vi "ExitApp (SubVI).vi"(8 "error in (no error)":errorcluster, 11 "Display Queue in":refnum<queue>) -> (0 "error out":errorcluster, 3 "Display Queue out":refnum<queue>)   [LabVIEW 2017]
uses:
  Controls/DisplayControl.ctl
  Controls/DisplayCommand.ctl
  Controls/UpdateMessageControl.ctl
  Controls/UpdateMessageCommand.ctl
  Controls/UpdateMenuCommand.ctl
  Controls/EnableDisableCommand.ctl
  Global 1.vi
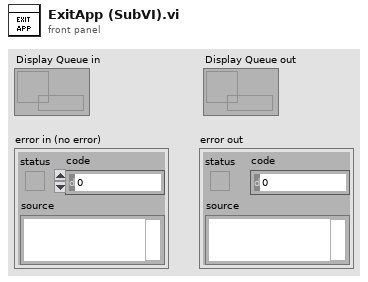
[diagram p1: front panel]
types:
  T1 = typedef "UpdateMessageControl.ctl" = cluster{"Command":T2, "Data":variant}
  T2 = typedef "UpdateMessageCommand.ctl" = enum16{"SystemCrash2", "SystemCrash1", "Welcome", "MainMenu", "PhoneNumberFailed", "PhoneNumberSuccess", "ParcelNumberSuccess", "ParcelNumbertFailed", "SessionTerminate", "SessionFinished", "Deposit", "DepositComplete", "Withdrawal", "WithdrawalComplete", "WithdrawalFailed"}
  T3 = typedef "DisplayControl.ctl" = cluster{"Command":T4, "Data":variant}
  T4 = typedef "DisplayCommand.ctl" = enum16{"Initialize", "Open/Close Parcel", "Enable/Disable Controls", "FocusCursor", "UpdateMessage", "UpdateMenus", "FinishOperation", "Exit", "CleanUserInput"}
  T5 = typedef "EnableDisableCommand.ctl" = enum16{"InitialSetup", "StartOperation", "EnableUserInput", "DisableUserInput", "EnableMenus", "DisableMenus"}
  T6 = typedef "UpdateMenuCommand.ctl" = enum16{"MainMenu", "NoMenu"}
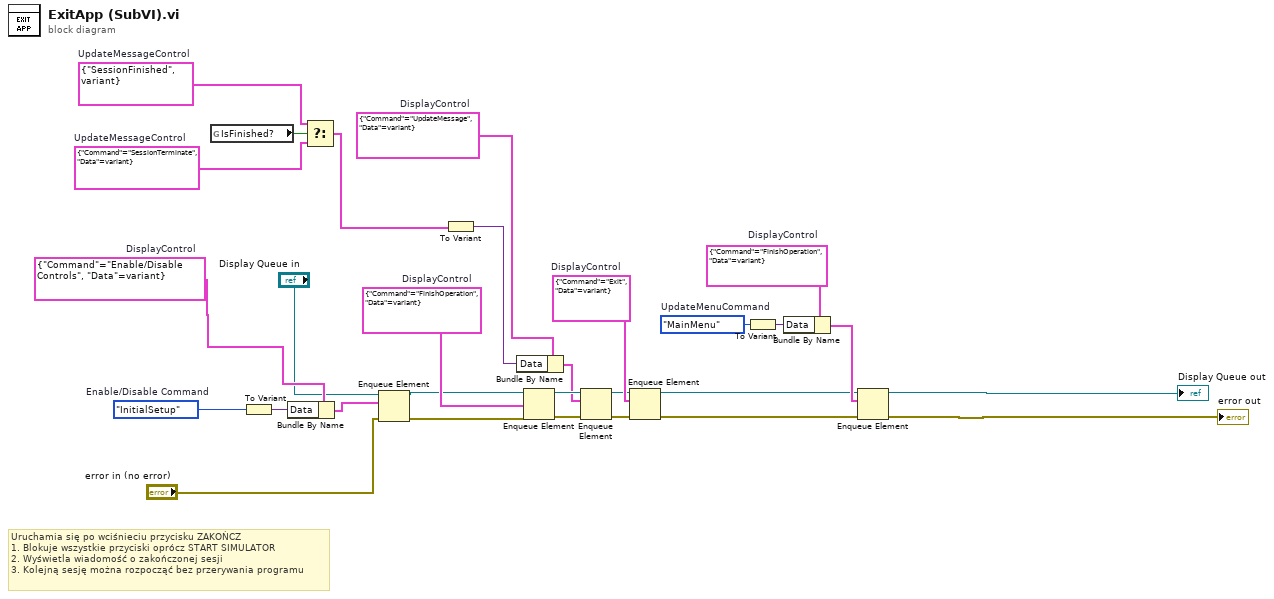
[diagram p0: block diagram]
diagram:
  w1 = T1 {"Command"=enum."SessionTerminate", "Data"=variant}  # UpdateMessageControl
  w11 = T3 {"Command"=enum."Enable/Disable Controls", "Data"=variant}  # DisplayControl
  w13 = EnableDisableCommand."InitialSetup"  # Enable/Disable Command
  w15 = T3 {"Command"=enum."FinishOperation", "Data"=variant}  # DisplayControl
  w20 = T3 {"Command"=enum."FinishOperation", "Data"=variant}  # DisplayControl
  w21 = UpdateMenuCommand."MainMenu"  # UpdateMenuCommand
  w2 = T1 {"Command"=enum."SessionFinished", "Data"=variant}  # UpdateMessageControl
  w24 = T3 {"Command"=enum."UpdateMessage", "Data"=variant}  # DisplayControl
  w29 = T3 {"Command"=enum."Exit", "Data"=variant}  # DisplayControl
  # "Uruchamia się po wciśnieciu przycisku ZAKOŃCZ\n1. Blokuje wszystkie przyciski oprócz START SIMULATOR\n2. Wyświetla wiadomość o zakończonej sesji\n3. Kolejną sesję można rozpocząć bez przerywania programu"
  n1 = global read "Global 1.vi" "IsFinished?"() -> (w4:bool)
  n2 = To Variant(anything=w13) -> (Variant=w14:variant)
  n3 = Bundle By Name(cluster=w11, "Data"=w14) -> (w12:T3)
  n4 = Select(t=w2, s=w4, f=w1) -> (s? t:f=w3:T1)
  n5 = Enqueue Element(queue="Display Queue in", element=w12, error in (no error)="error in (no error)") -> (queue out=w9:refnum<queue>, error out=w7:errorcluster)  [unwired: 1 in, 1 out]
  n6 = To Variant(anything=w3) -> (Variant=w23:variant)
  n7 = Bundle By Name(cluster=w24, "Data"=w23) -> (w22:T3)
  n8 = Enqueue Element(queue=w9, element=w15, error in (no error)=w7) -> (queue out=w27:refnum<queue>, error out=w26:errorcluster)  [unwired: 1 in, 1 out]
  n9 = Enqueue Element(queue=w27, element=w22, error in (no error)=w26) -> (queue out=w25:refnum<queue>, error out=w28:errorcluster)  [unwired: 1 in, 1 out]
  n10 = Enqueue Element(queue=w25, element=w29, error in (no error)=w28) -> (queue out=w17:refnum<queue>, error out=w16:errorcluster)  [unwired: 1 in, 1 out]
  n11 = To Variant(anything=w21) -> (Variant=w18:variant)
  n12 = Bundle By Name(cluster=w20, "Data"=w18) -> (w19:T3)
  n13 = Enqueue Element(queue=w17, element=w19, error in (no error)=w16) -> (queue out=→"Display Queue out":refnum<queue>, error out=→"error out":errorcluster)  [unwired: 1 in, 1 out]
